vi "fpga_LP2 Filter.vi"(0 "input data":fxp<+/-,32,5>, 1 "reset":bool, 5 "#Ch":fxp<+,5,5>=16.0, 9 "input valid":bool) -> (4 "output data":fxp<+/-,32,6>, 10 "output valid":bool, 14 "ready for input":bool)   [LabVIEW 2011, in "NI_EP_PMU_FPGA.lvlib"]
doc: "----------------------\n\nThis filter is configured as follows:\n\n<b>Filter Configuration</b>\nType: Single Rate\nStructure: FIR Direct Form\n\n<b>Input Data Type</b>\nType: fixed-point <±,32,5> [-1.600000E+1,1.600000E+1]:7.450581E-9\n\n<b>Output Data Type</b>\nType: fixed-point <±,32,6> [-3.200000E+1,3.200000E+1]:1.490116E-8\nRounding mode: Truncate\nOverflow mode: Wrap\n\n<b>Implementation</b>\nNumber of channels: 16\nMaximum input sampling rate per channel @ 40MHz: 11.737kHz\nGain processing: On Host\nMethod: Multiply-Accumulate\nNumber of multiply pipeline stages: 1\nMultiply register in: False\nNumber of adder levels per register: 2\nState memory: Block Memory\nCoefficient memory: Block Memory\n\n<b>Execution Mode</b>\nInside single-cycle Timed Loop\nThroughput: 213 cycles/sample\n\n<b>Estimated Resources</b>\nNumber of multiply-accumulate units: 1\nMultiply operation: I32.5 x I16.-4 => I48.6"
uses:
  <vilib>/addons/Electrical Power/PMU/NI_EP_PMU_FPGA.lvlib
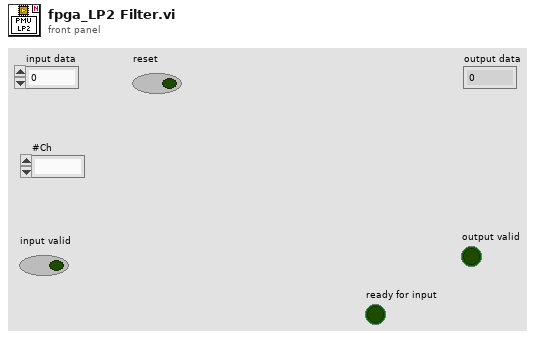
[diagram p1: front panel]
types:
  T1 = cluster{"WREn":bool, "WRAddr":fxp<+,12,12>, "RDAddr":fxp<+,12,12>, "BufWREn":bool, "BufWRAddr":fxp<+,12,12>, "firstRun":bool, "BufFiirstRun":bool}
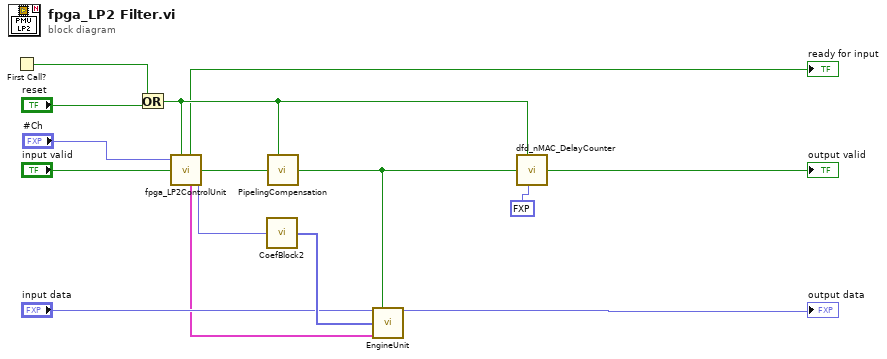
[diagram p0: block diagram]
diagram:
  n1 = First Call?() -> (First Call?: T/F=w12:bool)
  n2 = Or(x=w12, y="reset") -> (x .or. y?=w11:bool)
  n3 = call <vilib>:"fpga_LP2ControlUnit.vi"("#Ch"="#Ch", "reset"=w11, "input valid"="input valid") -> ("ready for input"=→"ready for input":bool, "output valid"=w14:bool, "opState"=w3:T1, "coefRDAddr"=w2:fxp<+,8,8>)  [unwired: 3 in]
  n4 = call "CoefBlock2"("coefAddr"=w2) -> ("coefficients"=w6:fxp<+/-,17,-3>[])  [unwired: 8 in]
  n5 = call "PipelingCompensation"("reset"=w11, "data in"=w14) -> ("data out"=w5:bool)  [unwired: 7 in]
  n6 = call "EngineUnit"("input data"="input data", "ACC_Load"=w5, "coefficients"=w6, "opState"=w3) -> ("output data"=→"output data":fxp<+/-,32,6>)  [unwired: 11 in]
  n7 = call "dfd_nMAC_DelayCounter.vi"("reset"=w11, "data in"=w5, "#delay"=fxp<+,8,8> 213.0 ("#TPPM")) -> ("data out"=→"output valid":bool)  [unwired: 6 in]
